vi "I2C_read.vi"(10 "Min time SCL Low":u32 caption="Low", 11 "Min Time SCL High":u32 caption="High") -> (3 "reversed array":bool[](array[boolean]))   [LabVIEW 2019]
uses:
  <vilib>/rvi/Emulation/niFpgaGetClockAttributes.vi
  <vilib>/rvi/Emulation/niFpgaSctlEmulationGetInTimedLoop.vi
  <vilib>/rvi/Emulation/niFpgaEmulationReportErrorSimple.vi
  <vilib>/rvi/eio/common/nirviEmuTemplateMethod_errors.vi
  <vilib>/rvi/Emulation/niFpgaCriticalErrorInLSC.vi
  <vilib>/eio/EIONode/EIONode.xnode
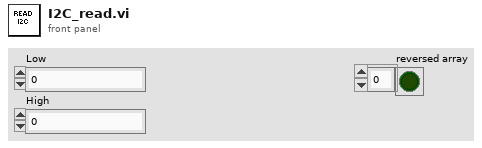
[diagram p1: front panel]
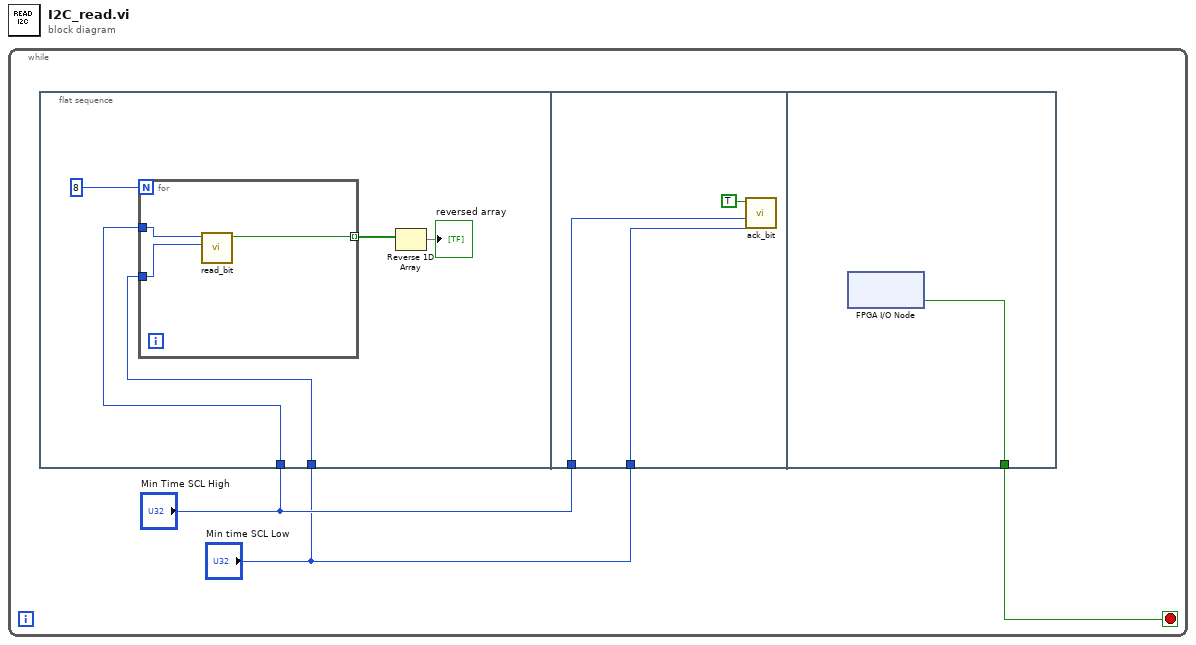
[diagram p0: block diagram]
diagram:
  n1 = while {
    stop <- w1 stop-if-true
    n2 = flat-sequence {
      tunnel: "Min Time SCL High" -> [w7]
      tunnel: "Min time SCL Low" -> [w6]
      tunnel: "Min time SCL Low" -> [w12]
      tunnel: "Min Time SCL High" -> [w13]
      tunnel: [w15] -> w1
      frame #0 {
        n3 = for {
          N: 8 -> [_]
          tunnel: w7 -> [w11]
          tunnel: w6 -> [w10]
          tunnel: [w9] -> w5 mode=indexing
          n4 = call "read_bit.vi"("Min time SCL low"=w10, "Min Time SCL high"=w11) -> ("Data bit"=w9:bool)  [unwired: 9 in]
        }
        n5 = Reverse 1D Array(array=w5) -> (reversed array=→"reversed array":bool[])
      }
      frame #1 {
        n6 = call "ack_bit.vi"("Min time SCL Low"=w12, "Min Time SCL High"=w13, "ack"=TRUE) -> ()  [unwired: 9 in]
      }
      frame #2 {
        n7 = xnode "FPGA I/O Node"() -> ("SDA"=w15:bool)  [unwired: 1 in, 1 out]
      }
    }
  }
